vi "Simulate Mosaic.vi"() -> ()   [LabVIEW 2018]
panel:
  in  "input cluster":T1={"X Axis"={"Start [mm]"=0.0, "Steps [pts]"=3.3, "End [mm]"=0.0}, "Y Axis"={"Start [mm]"=0.0, "Steps [pts]"=3.3, "End [mm]"=0.0}, "Scan Pattern"=enum."Uni-directional", "Overlap Options"={"Overlap Type"=enum."No Overlap", "Percent Overlap"=0, "Justify"=enum."Start"}}
  out "Array":cluster{"X":dbl, "Y":dbl}[](array[cluster])
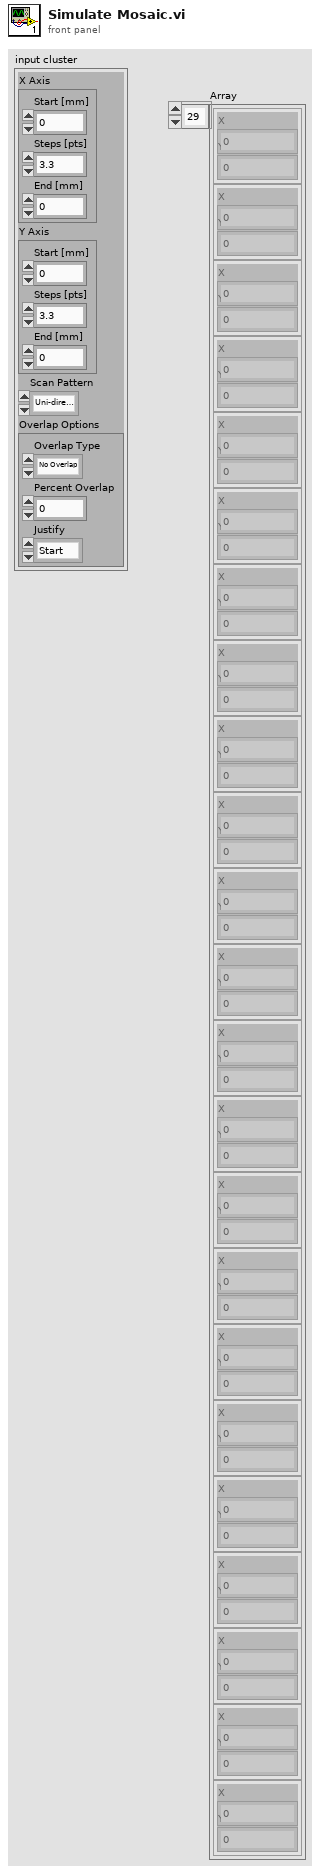
[diagram p1: front panel]
types:
  T1 = cluster{"X Axis":cluster{"Start [mm]":dbl, "Steps [pts]":dbl, "End [mm]":dbl}, "Y Axis":cluster{"Start [mm]":dbl, "Steps [pts]":dbl, "End [mm]":dbl}, "Scan Pattern":enum16{"Uni-directional", "Bi-Directional", "Spiral Out", "Spiral In"}, "Overlap Options":cluster{"Overlap Type":enum16{"No Overlap", "X Only", "Y Only", "X and Y"}, "Percent Overlap":u8, "Justify":enum16{"Start", "Center", "End"}}}
  T2 = cluster{"Start [mm]":dbl, "Steps [pts]":dbl, "End [mm]":dbl}
  T3 = cluster{"Overlap Type":enum16{"No Overlap", "X Only", "Y Only", "X and Y"}, "Percent Overlap":u8, "Justify":enum16{"Start", "Center", "End"}}
  T4 = enum16{"Uni-directional", "Bi-Directional", "Spiral Out", "Spiral In"}
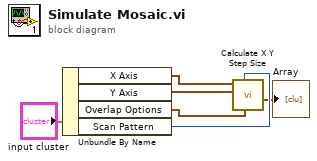
[diagram p0: block diagram]
diagram:
  n1 = Unbundle By Name("input cluster") -> ("X Axis"=w6:T2, "Y Axis"=w5:T2, "Overlap Options"=w4:T3, "Scan Pattern"=w3:T4)
  n2 = call "Calculate X Y Step Size.vi"("Overlap Options"=w4, "Scan Pattern"=w3, "Y Axis"=w5, "X Axis"=w6) -> ("Array"=→"Array":cluster{"X":dbl, "Y":dbl}[])  [unwired: 4 in, 3 out]
